vi "calculations.vi"(6 "pi":dbl, 9 "AGE Initial \nDiameter [in]":dbl, 10 "AGE Effective Width [mm]":dbl, 11 "AGE Fiber \nSurface Area [m^2]":dbl) -> (1 "l_w":dbl, 2 "n":dbl, 3 "age_od":dbl, 4 "sh_r":dbl)   [LabVIEW 2016]
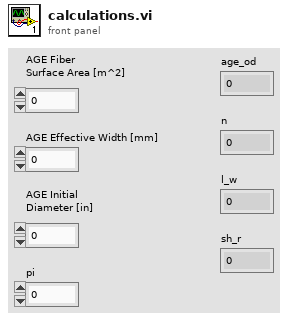
[diagram p1: front panel]
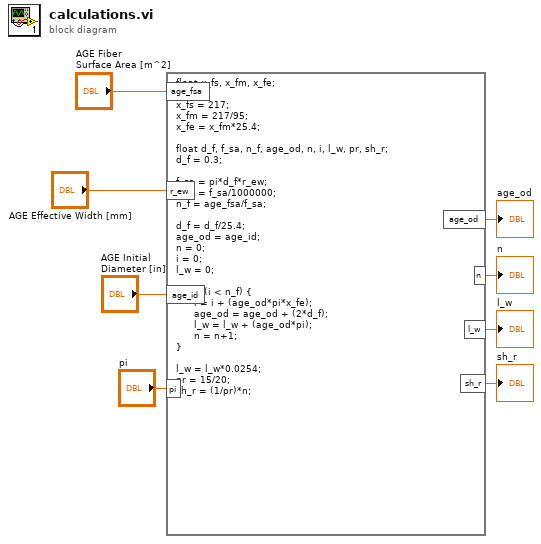
[diagram p0: block diagram]
diagram:
  n1 = formula code="float x_fs, x_fm, x_fe;\n\nx_fs = 217;\nx_fm = 217/95;\nx_fe = x_fm*25.4;\n\nfloat d_f, f_sa, n_f, age_od, n, i, l_w, pr, sh_r;\nd_f = 0.3;\n\nf_sa = pi*d_f*r_ew;\nf_sa = f_sa/1000000;\nn_f = age_fsa/f_sa;\n\nd_f = d_f/25.4;\nage_od = age_id;\nn = 0;\ni = 0;\nl_w = 0;\n\nwhile (i < n_f) {\n      i = i + (age_od*pi*x_fe);\n      age_od = age_od + (2*d_f);\n      l_w = l_w + (age_od*pi);\n      n = n+1; \n}\n\nl_w = l_w*0.0254; \npr = 15/20;\nsh_r = (1/pr)*n;"("age_fsa"="AGE Fiber \nSurface Area [m^2]", "r_ew"="AGE Effective Width [mm]", "age_id"="AGE Initial \nDiameter [in]", "pi"="pi") -> ("sh_r"=→"sh_r":dbl, "n"=→"n":dbl, "age_od"=→"age_od":dbl, "l_w"=→"l_w":dbl)
